vi "Get LTS Max Stage Acceleration.vi"(8 "error in (no error)":errorcluster, 10 "Cluster in":T1, 11 "LTS Reference In":refnum<k24>) -> (0 "error out":errorcluster, 1 "AccelerationMaximum":dbl, 2 "Cluster out":T1, 3 "LTS Reference Out":refnum<k24>)   [LabVIEW 2014]
uses:
  Controls/Translation Stage Cluster.ctl
  C:/Projects/Serial Sectioning OCT - TortoiseGIT/SerialSectOCT/Software/Thorlabs.MotionControl.Controls.dll
  Thorlabs.MotionControl.Controls.dll
  C:/Projects/Serial Sectioning OCT - TortoiseGIT/SerialSectOCT/Software/Thorlabs.MotionControl.IntegratedStepperMotorsCLI.dll
  Thorlabs.MotionControl.IntegratedStepperMotorsCLI.dll
  C:/Projects/Serial Sectioning OCT - TortoiseGIT/SerialSectOCT/Software/Thorlabs.MotionControl.GenericMotorCLI.dll
  Thorlabs.MotionControl.GenericMotorCLI.dll
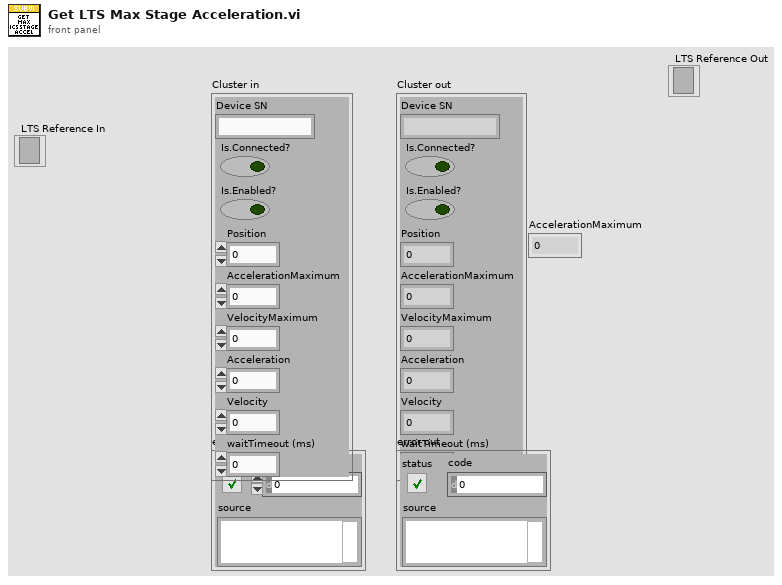
[diagram p1: front panel]
types:
  T1 = typedef "Translation Stage Cluster.ctl" = cluster{"Device SN":string, "Is.Connected?":bool, "Is.Enabled?":bool, "Position":dbl, "AccelerationMaximum":dbl, "VelocityMaximum":dbl, "Acceleration":dbl, "Velocity":dbl, "waitTimeout (ms)":i32}
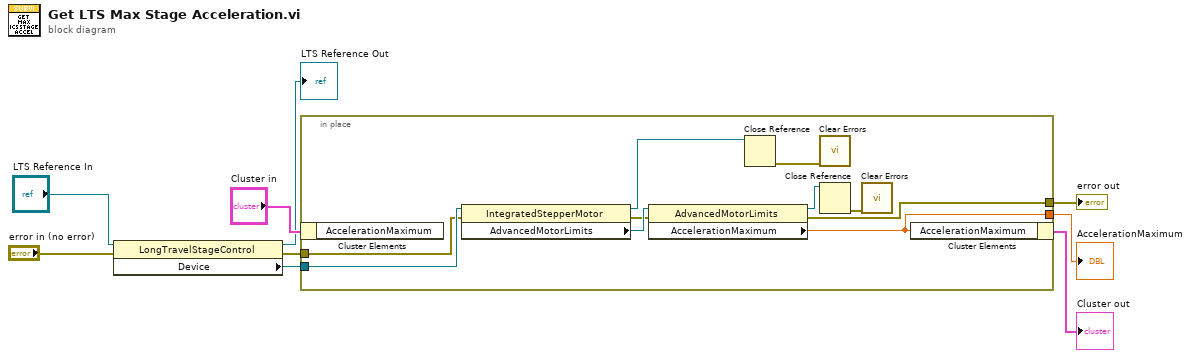
[diagram p0: block diagram]
diagram:
  n1 = property class="LongTravelStageControl"(reference="LTS Reference In", error in="error in (no error)") -> (reference out=→"LTS Reference Out":refnum<k24>, error out=w4:errorcluster, "Device"=w1:refnum<k24>)
  n2 = in-place {
    in-place-border: [w13] -> w7
    in-place-border: w1 -> [w12]
    in-place-border: w4 -> [w11]
    in-place-border: [w10] -> w6
    n3 = in-place-cluster #1("Cluster in") -> ()  [unwired: 1 out]
    n4 = property class="IntegratedStepperMotor"(reference=w12, error in=w11) -> (reference out=w16:refnum<k24>, error out=w18:errorcluster, "AdvancedMotorLimits"=w19:refnum<k24>)
    n5 = property class="AdvancedMotorLimits"(reference=w19, error in=w18) -> (reference out=w14:refnum<k24>, error out=w13:errorcluster, "AccelerationMaximum"=w10:dbl)
    n6 = Close Reference(reference=w16) -> (error out=w17:errorcluster)  [unwired: 1 in]
    n7 = call <vilib>:"Clear Errors.vi"("error in (no error)"=w17) -> ()  [unwired: 5 in, 2 out]
    n8 = Close Reference(reference=w14) -> (error out=w15:errorcluster)  [unwired: 1 in]
    n9 = call <vilib>:"Clear Errors.vi"("error in (no error)"=w15) -> ()  [unwired: 5 in, 2 out]
    n10 = in-place-cluster #1("AccelerationMaximum"=w10) -> (→"Cluster out":T1)
  }
  "error out" <- w7
  "AccelerationMaximum" <- w6
